vi "SubVI_CalculaIMC.vi"(3 "error in":errorcluster, 4 "Altura":dbl format="%#_13g", 5 "Peso":dbl format="%#_13g") -> (0 "error out":errorcluster, 1 "IMC em string":string, 2 "IMC":dbl format="%#.2f")   [LabVIEW 2023]
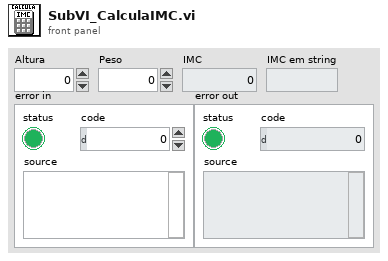
[diagram p1: front panel]
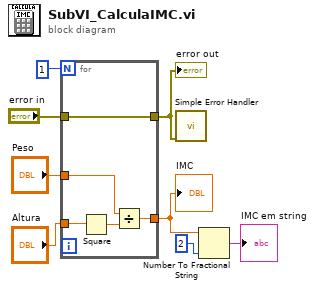
[diagram p0: block diagram]
diagram:
  n1 = for {
    N: 1 -> [_]
    tunnel: "Altura" -> [w13]
    tunnel: "Peso" -> [w12]
    tunnel: [w10] -> w2
    tunnel: "error in" -> [w9]
    tunnel: [w9] -> w4
    n2 = Square(x=w13) -> (x^2=w11:dbl)
    n3 = Divide(x=w12, y=w11) -> (x/y=w10:dbl)
  }
  "IMC" <- w2
  "error out" <- w4
  n4 = call <vilib>:"Simple Error Handler.vi"("error in (no error)"=w4) -> ()  [unwired: 4 in, 5 out]
  n5 = Number To Fractional String(number=w2, precision (6)=i16 2) -> (F-format string=→"IMC em string":string)  [unwired: 2 in]
